vi "SeekForward_171213.vi"(6 "Y in":i32[](array[numeric]), 9 "Y out 4":i32[](array[numeric]), 10 "Seek Forward Button":bool, 11 "Boolean in":refnum<vi>) -> (2 "Y out":i32[](array[numeric]), 3 "Y out 3":i32[](array[numeric]))   [LabVIEW 2016]
uses:
  Globaltracker.vi
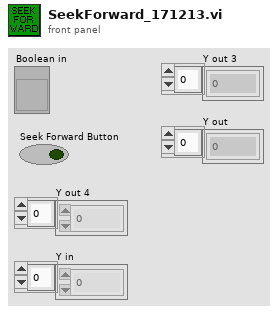
[diagram p1: front panel]
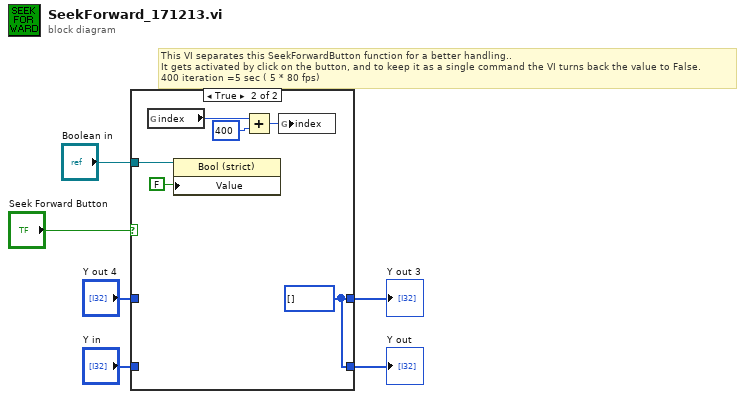
[diagram p0: block diagram]
diagram:
  # "This VI separates this SeekForwardButton function for a better handling..\nIt gets activated by click on the button, and to keep it as a single command the VI turns back the value to False. \n400 iteration =5 sec ( 5 * 80 fps)"
  n1 = case shown="True" "Seek Forward Button" {
    tunnel: "Y out 4" -> [w8 _]
    tunnel: [w8 w12] -> w3
    tunnel: "Y in" -> [w7 _]
    tunnel: [w7 w12] -> w5
    tunnel: "Boolean in" -> [_ w9]
    frame False {
    }
    frame True {
      w12 = i32[] [] ("Y out")
      n2 = global read "Globaltracker.vi" "index"() -> (w11:i16)
      n3 = property class="Bool (strict)"(reference=w9, "Value"=FALSE ("Seek Forward Button")) -> ()  [unwired: 1 in, 2 out]
      n4 = Add(x=w11, y=400) -> (x+y=w10:i32)
      n5 = global write "Globaltracker.vi" "index"(w10) -> ()
    }
  }
  "Y out" <- w5
  "Y out 3" <- w3
